vi "TestCOMxsquarearray.vi"() -> ()   [LabVIEW 2012]
panel:
  out "数据":dbl[][](array[numeric])
  in  "数组":dbl[][](array[numeric])
  in  "xsquare.IClass1":refnum<k7>
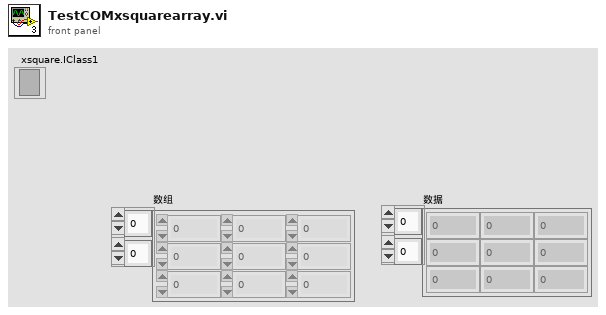
[diagram p1: front panel]
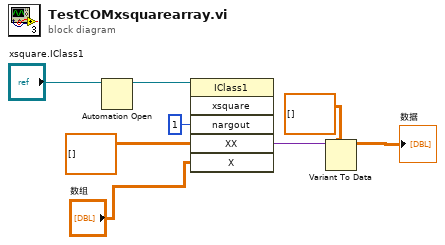
[diagram p0: block diagram]
diagram:
  n1 = Automation Open(Automation Refnum="xsquare.IClass1") -> (Automation Refnum=w6:refnum<k7>)  [unwired: 3 in, 1 out]
  n2 = invoke class="IClass1" method="xsquare"(reference=w6, "nargout"=1, "XX"=dbl[][] [], "X"="数组") -> ("XX"=w8:variant)  [unwired: 2 in, 5 out]
  n3 = Variant To Data(type=dbl[][] [], Variant=w8) -> (data=→"数据":dbl[][])  [unwired: 1 in, 1 out]
